vi "Create File Sink.vi"(8 "error in (no error)":errorcluster, 11 "Path":path) -> (0 "error out":errorcluster)   [LabVIEW 2020, in "LV Logging.lvlib"]
uses:
  LV Logging.lvlib
  File Sink/File Sink.lvclass
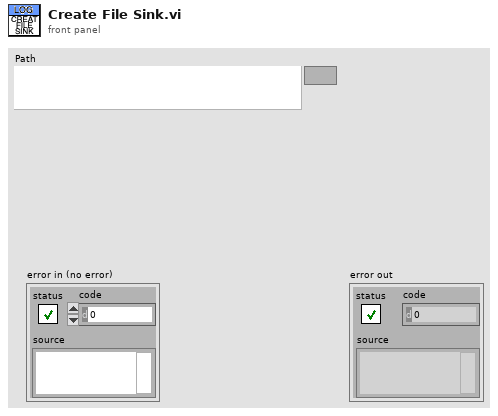
[diagram p1: front panel]
types:
  T1 = enum16{"Init", "Get Logger", "Register Sink", "Set Global Debug Level", "Get Sinks"}
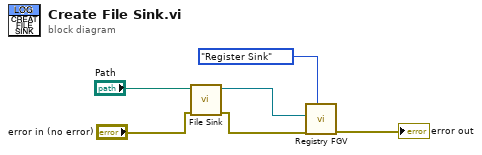
[diagram p0: block diagram]
diagram:
  n1 = call "File Sink.vi"("error in (no error)"="error in (no error)", "File Path"="Path") -> ("error out"=w2:errorcluster, "File Sink out"=w4:refnum<class "File Sink.lvclass">)  [unwired: 8 in]
  n2 = call "Registry FGV.vi"("State (Get Logger)"=T1."Register Sink", "error in (no error)"=w2, "Sink"=w4) -> ("error out"=→"error out":errorcluster)  [unwired: 5 in, 3 out]
